vi "Module Cleanup.vi"(8 "error in (no error)":errorcluster, 11 "Telemetry Command Module in":refnum<class "Telemetry Command Module.lvclass">) -> (0 "error out":errorcluster, 3 "Telemetry Command Module out":refnum<class "Telemetry Command Module.lvclass">)   [LabVIEW 2020, in "VolatusGUI.lvlib" / "Telemetry Command Module.lvclass"]
uses:
  Telemetry Command Module.lvclass
  Telemetry Command Module.lvclass/Telemetry Command Module.ctl
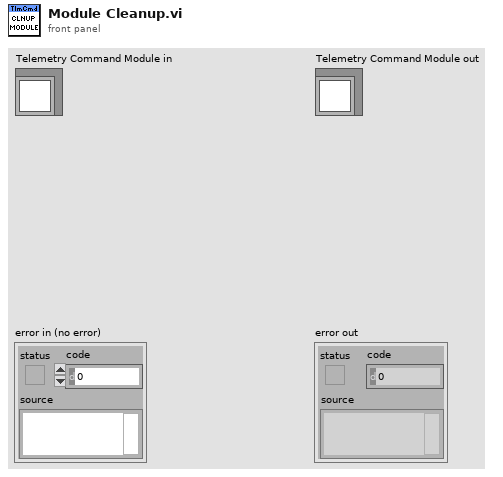
[diagram p1: front panel]
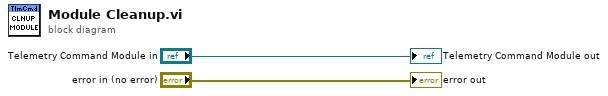
[diagram p0: block diagram]
diagram:
  "error out" <- "error in (no error)"
  "Telemetry Command Module out" <- "Telemetry Command Module in"
